vi "Read FP Source Dir.vi"(9 "RasPi Compiler in":refnum<class "RasPi Compiler.lvclass">) -> (3 "RasPi Compiler out":refnum<class "RasPi Compiler.lvclass">, 4 "FP Source Dir":path)   [LabVIEW 2014, in "RasPi Compiler.lvclass"]
uses:
  RasPi Compiler.lvclass
  RasPi Compiler.lvclass/RasPi Compiler.ctl
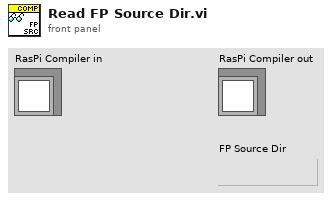
[diagram p1: front panel]
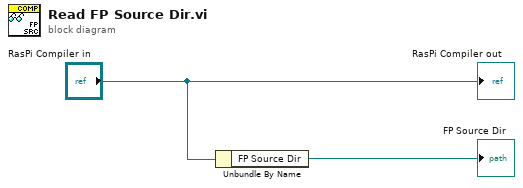
[diagram p0: block diagram]
diagram:
  n1 = Unbundle By Name("RasPi Compiler in") -> ("FP Source Dir"=→"FP Source Dir":path)
  "RasPi Compiler out" <- "RasPi Compiler in"
